vi "NI 5413 trigger control.vi"(7 "FGEN Resource Name":refnum<k15>, 9 "Amplitude":dbl=2.0 format="%0_3g", 10 "Frequency":dbl=1000000.0 format="%.2p", 11 "Standard Waveform":u16(ring) items=["Sine", "Square", "Triangle", "Ramp Up", "Ramp Down", "DC", "Noise"]) -> (0 "error out":errorcluster, 3 "Instrument Handle Out":refnum<k15>)   [LabVIEW 2020]
doc: "This example shows how to use Standard Function mode. This is a basic example that shows the smallest amount of code necessary to generate a standard waveform."
uses:
  <instrlib>/niFgen/niFgen.llb/niFgen Output Mode.ctl
panel:
  # "Overview: Demonstrates how to configure an NI Signal Source to generate a basic standard function.\nSoftware Requirements: NI-FGEN\nHardware Requirements: PXI-5401, PCI-5401, PXI-5402, PCI-5402, PXI-5406, PCI-5406, PXI-5411, PCI-5411, AT-5411, PXI-5412, PCI-5412, PXIe-5413, PXI-5421, PCI-5421, PXI-5422, PXIe-5423, PXI-5431, PCI-5431, PXIe-5433, PXI-5441, NI PXIe-5442, NI PXIe-5450, or NI PXIe-5451 \nInstructions:\n1. Select the FGEN Resource Name as configured in the Measurement & Automation Explorer.\n2. Select the Standard Waveform to be generated.\n3. Specify the desired Frequency for the waveform.\n4. Select to Amplitude of the waveform.\n5. Run the VI.\n6. Click Stop to stop the VI."
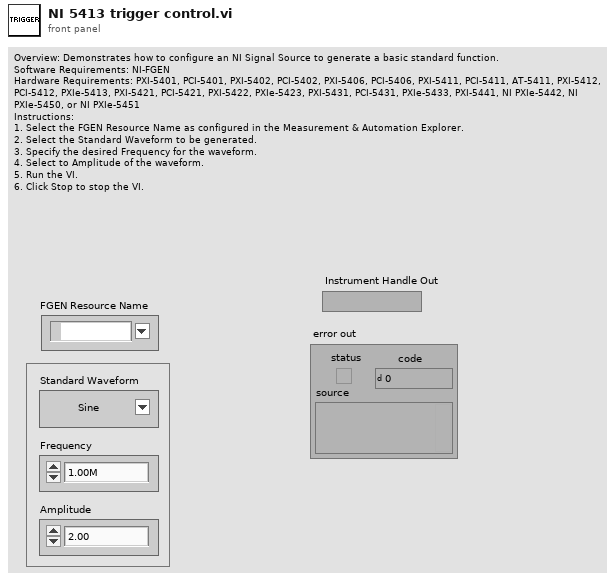
[diagram p1: front panel]
types:
  T1 = typedef "niFgen Output Mode.ctl" = u32
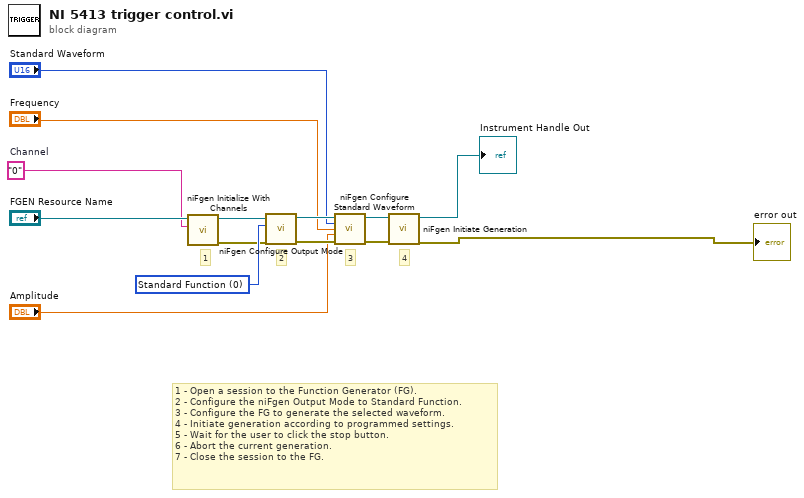
[diagram p0: block diagram]
diagram:
  w3 = "0"  # Channel
  w14 = T1 0 items=["Standard Function", "Frequency List", "Arbitrary Waveform", "Arbitrary Sequence", "Script"] ("output mode")
  # "4"
  # "3"
  # "2"
  # "1"
  # "1 - Open a session to the Function Generator (FG).\n2 - Configure the niFgen Output Mode to Standard Function.\n3 - Configure the FG to generate the selected waveform.\n4 - Initiate generation according to programmed settings.\n5 - Wait for the user to click the stop button.\n6 - Abort the current generation.\n7 - Close the session to the FG."
  n1 = call <instrlib>:"niFgen Initialize With Channels.vi"("Channel Name"=w3, "Resource Name"="FGEN Resource Name") -> ("error out"=w4:errorcluster, "Instrument Handle Out"=w5:refnum<k15>)  [unwired: 8 in]
  n2 = call <instrlib>:"niFgen Configure Output Mode.vi"("error in (no error)"=w4, "Output Mode (default: 0=Standard Function)"=w14, "Instrument Handle"=w5) -> ("error out"=w10:errorcluster, "Instrument Handle Out"=w11:refnum<k15>)  [unwired: 6 in]
  n3 = call <instrlib>:"niFgen Configure Standard Waveform.vi"("Instrument Handle"=w11, "Waveform"="Standard Waveform", "Frequency"="Frequency", "Amplitude"="Amplitude", "error in (no error)"=w10) -> ("Instrument Handle Out"=w12:refnum<k15>, "error out"=w13:errorcluster)  [unwired: 9 in]
  n4 = call <instrlib>:"niFgen Initiate Generation.vi"("error in (no error)"=w13, "Instrument Handle"=w12) -> ("error out"=→"error out":errorcluster, "Instrument Handle Out"=→"Instrument Handle Out":refnum<k15>)  [unwired: 8 in]
